vi "Get Thread ID Pool.vi"(11 "Plugin in":refnum<class "Plugin.lvclass">) -> (2 "Thread ID Pool":refnum<class "ID Pool.lvclass">, 3 "Plugin out":refnum<class "Plugin.lvclass">)   [LabVIEW 2017, in "DSF Core.lvlib" / "Plugin.lvclass"]
uses:
  Plugin.lvclass
  Thread Pool/ID Pool.lvclass
  Plugin.lvclass/Plugin.ctl
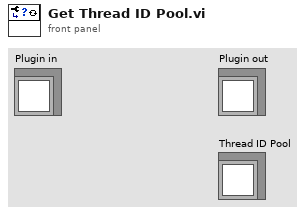
[diagram p1: front panel]
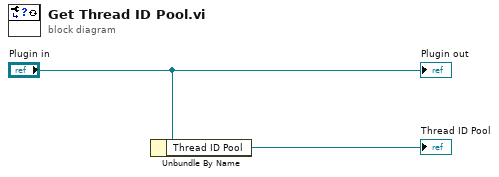
[diagram p0: block diagram]
diagram:
  n1 = Unbundle By Name("Plugin in") -> ("Thread ID Pool"=→"Thread ID Pool":refnum<class "ID Pool.lvclass">)
  "Plugin out" <- "Plugin in"
